vi "MFC WR.vi"() -> ()   [LabVIEW 2014]
panel:
  out "Overall":u32
  out "Timing":u32[](array[numeric])
  out "MFC PV":u8[](array[numeric])
  out "MFC out":u8[](array[numeric])
  out "Numeric":i32
  in  "Out Array":u8[](array[numeric])=[65, 48, 48, 48, 48, 48, 13, 65, 48, 48, 48, 48, 48, 13, 67, 48, 48, 48, 48, 48, 13, 68, 48, 48, 48, 48, 48, 13, 69, 48, 48, 48, 48, 48, 13, 70, 48, 48, 48, 48, 48, 13, 71, 48, 48, 48, 48, 48, 13, 72, 48, 48, 48, 48, 48, 13, 73, 48, 48, 48, 48, 48, 13]
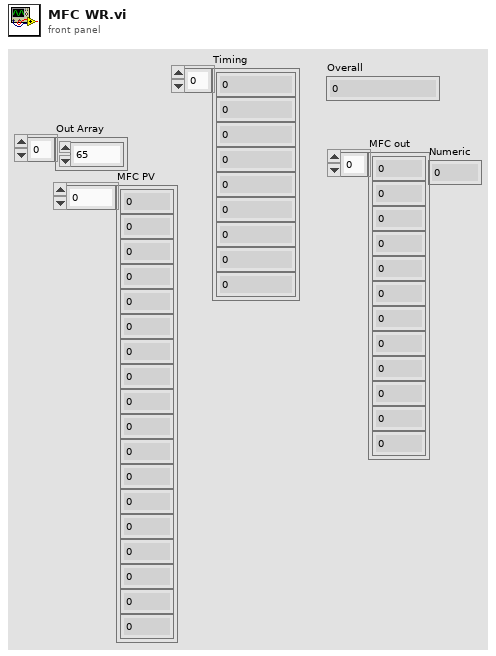
[diagram p1: front panel]
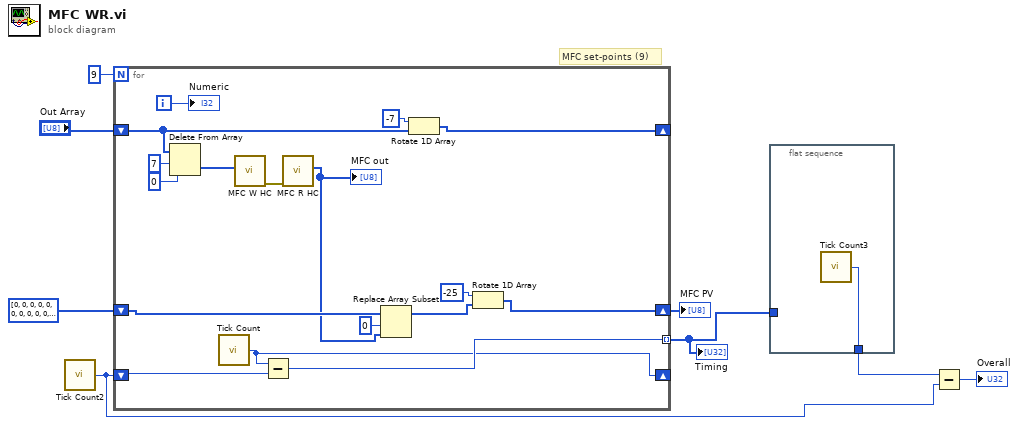
[diagram p0: block diagram]
diagram:
  # "MFC set-points (9)"
  n1 = call "Tick Count2"() -> ("Tick Count(Ticks)"=w4:u32)
  n2 = for {
    N: 9 -> [_]
    shift-right: [w23] -> _
    shift-left: "Out Array" -> [w24]
    shift-right: [w14] -> w5
    shift-left: u8[] [0, 0, 0, 0, 0, 0, 0, 0, 0, 0, 0, 0, 0, 0, 0, 0, 0, 0, 0, 0, 0, 0, 0, 0, 0, 0, 0, 0, 0, 0, 0, 0, 0, 0, 0, 0, 0, 0, 0, 0, 0, 0, 0, 0, 0, 0, 0, 0, 0, 0, 0, 0, 0, 0, 0, 0, 0, 0, 0, 0, 0, 0, 0, 0, 0, 0, 0, 0, 0, 0, 0, 0, 0, 0, 0, 0, 0, 0, 0, 0, 0, 0, 0, 0, 0, 0, 0, 0, 0, 0, 0, 0, 0, 0, 0, 0, 0, 0, 0, 0, 0, 0, 0, 0, 0, 0, 0, 0, 0, 0, 0, 0, 0, 0, 0, 0, 0, 0, 0, 0, 0, 0, 0, 0, 0, 0, 0, 0, 0, 0, 0, 0, 0, 0, 0, 0, 0, 0, 0, 0, 0, 0, 0, 0, 0, 0, 0, 0, 0, 0, 0, 0, 0, 0, 0, 0, 0, 0, 0, 0, 0, 0, 0, 0, 0, 0, 0, 0, 0, 0, 0, 0, 0, 0, 0, 0, 0, 0, 0, 0, 0, 0, 0, 0, 0, 0, 0, 0, 0, 0, 0, 0, 0, 0, 0, 0, 0, 0, 0, 0, 0, 0, 0, 0, 0, 0, 0, 0, 0, 0, 0, 0, 0, 0, 0, 0, 0, 0, 0, 0, 0, 0, 0, 0, 0] -> [w17]
    tunnel: [w10] -> w1 mode=indexing
    shift-right: [w9] -> _
    shift-left: w4 -> [w11]
    i -> [w19]
    n3 = Delete From Array(array=w24, length=7, index=0) -> (deleted portion=w18:u8[])  [unwired: 1 out]
    n4 = call "Tick Count"() -> ("Tick Count(Ticks)"=w9:u32)
    n5 = call "MFC W HC.vi"("Byte array"=w18) -> ("error out"=w20:errorcluster)  [unwired: 10 in]
    n6 = Subtract(x=w9, y=w11) -> (x-y=w10:u32)
    n7 = call "MFC R HC.vi"("error in"=w20) -> ("MFC out"=w12:u8[])  [unwired: 8 in, 1 out]
    "MFC out" <- w12
    n8 = Replace Array Subset(array=w17, new element=w12, index=0) -> (w15:u8[])
    n9 = Rotate 1D Array(1:w24, 2:-7 ("n")) -> (0:w23:u8[])
    n10 = Rotate 1D Array(1:w15, 2:-25 ("n")) -> (0:w14:u8[])
    "Numeric" <- w19
  }
  "MFC PV" <- w5
  "Timing" <- w1
  n11 = flat-sequence {
    tunnel: [w26] -> w3
    tunnel: w1 -> [_]
    frame #0 {
      n12 = call "Tick Count3"() -> ("Tick Count(Ticks)"=w26:u32)
    }
  }
  n13 = Subtract(x=w3, y=w4) -> (x-y=→"Overall":u32)
